vi "Image Process By VBAI.vi"(8 "error in":errorcluster, 11 "VBAI":cluster{"New Image":T1, "VBAI Session Out":T2}) -> (0 "error out":errorcluster, 1 "Defect identify data":cluster{"Image":T1, "Measure Report":string}, 2 "Result":bool, 3 "Session Out":T2, 4 "缺陷数量":string, 5 "Image":T1(plugin-control))   [LabVIEW 2018]
uses:
  <vilib>/userdefined/High Color/VBAIInterface.ctl
  <vilib>/vision/Image Controls.llb/IMAQ Image.ctl
panel:
  out "Measurement Report":string
  out "Report Text":string
  out "String Measurement":string
  out "Inspection Status":bool
  out "New Image Available":bool
  out "Step Results":T3(array[cluster]) {"Numeric Measurement" format="%.2f"}
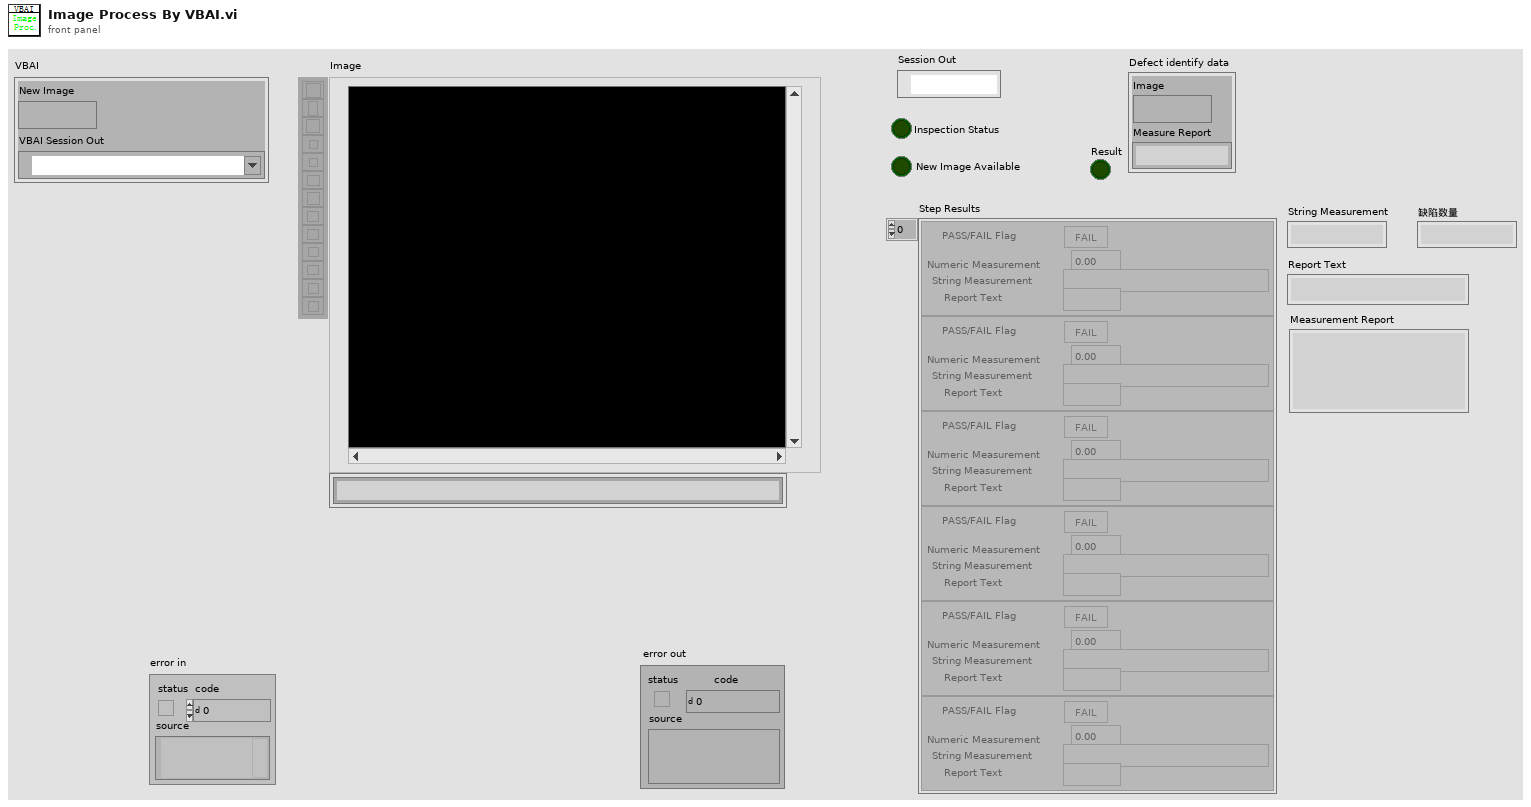
[diagram p1: front panel]
types:
  T1 = typedef "IMAQ Image.ctl" = refnum<image>
  T2 = typedef "VBAIInterface.ctl" = refnum<k21>
  T3 = cluster{"PASS/FAIL Flag":bool, "Numeric Measurement":dbl, "String Measurement":string, "Report Text":string}[]
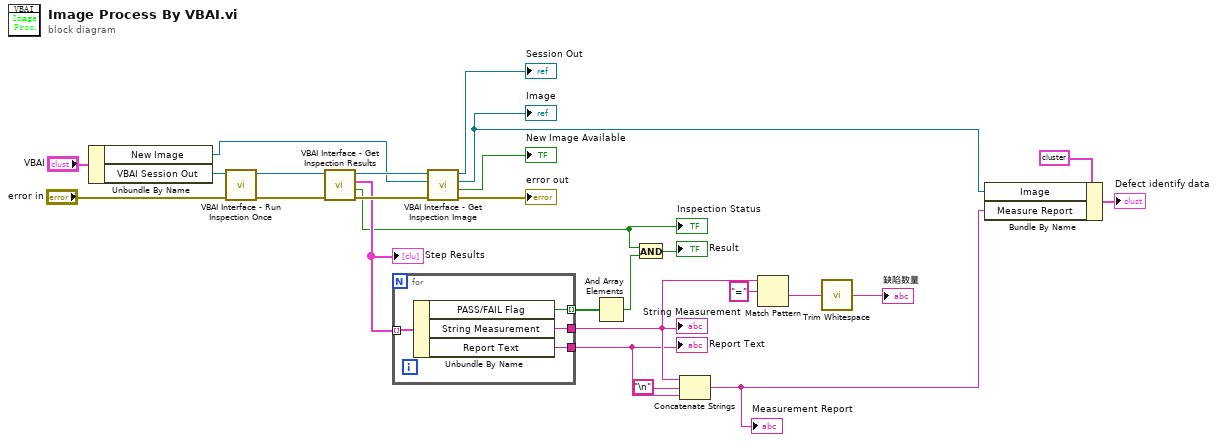
[diagram p0: block diagram]
diagram:
  n1 = Unbundle By Name("VBAI") -> ("New Image"=w2:T1, "VBAI Session Out"=w1:T2)
  n2 = call <vilib>:"VBAI Interface - Run Inspection Once.vi"("error in"="error in", "Session In"=w1) -> ("error out"=w20:errorcluster, "Session Out"=w21:T2)  [unwired: 8 in]
  n3 = call <vilib>:"VBAI Interface - Get Inspection Results.vi"("error in"=w20, "Session In"=w21) -> ("error out"=w25:errorcluster, "Inspection Status"=w15:bool, "Step Results"=w18:T3, "Session Out"=w26:T2)  [unwired: 3 in, 3 out]
  "Step Results" <- w18
  "Inspection Status" <- w15
  n4 = for {
    tunnel: w18 -> [w30] mode=indexing
    tunnel: [w29] -> w17 mode=indexing
    tunnel: [w28] -> w10
    tunnel: [w27] -> w9
    n5 = Unbundle By Name(w30) -> ("PASS/FAIL Flag"=w29:bool, "String Measurement"=w28:string, "Report Text"=w27:string)
  }
  "String Measurement" <- w10
  "Report Text" <- w9
  n6 = call <vilib>:"VBAI Interface - Get Inspection Image.vi"("error in"=w25, "Image Dest"=w2, "Session In"=w26) -> ("error out"=→"error out":errorcluster, "New Image Available"=→"New Image Available":bool, "Image Dst Out"=w5:T1, "Session Out"=→"Session Out":T2)  [unwired: 5 in]
  "Image" <- w5
  n7 = And Array Elements(Boolean array=w17) -> (logical AND=w16:bool)
  n8 = And(x=w15, y=w16) -> (x .and. y?=→"Result":bool)
  n9 = Concatenate Strings(w10, "\n", w9) -> (w6:string)
  "Measurement Report" <- w6
  n10 = Match Pattern(string=w10, regular expression="=" ("正则表达式")) -> (after substring=w12:string)  [unwired: 1 in, 3 out]
  n11 = call <vilib>:"Trim Whitespace.vi"("string"=w12) -> ("trimmed string"=→"缺陷数量":string)  [unwired: 1 in]
  n12 = Bundle By Name(cluster=cluster{"Image":T1, "Measure Report":string} {"Image"="remote image 00000000125D049C", "Measure Report"=""} ("Defect Identify data"), "Image"=w5, "Measure Report"=w6) -> (→"Defect identify data":cluster{"Image":T1, "Measure Report":string})
